vi "Process.vi"(9 "process sync":refnum<notifier>, 10 "TopLevel":refnum<class "TopLevel.lvclass">, 11 "DLP2 in":refnum<class "DLP2.lvclass">) -> ()   [LabVIEW 2022 SP3, in "DLP2.lvclass"]
doc: "Developed by Kevin Thompson\nkevin@thompsonengineering.net\n\nCopyright 2018\nThompson Engineering, LLC"
uses:
  DLP2.lvclass
  DataTypes/Read Data--cluster.ctl
  TopLevel/TopLevel.lvclass
  DataTypes/Process - AppData--cluster.ctl
  DataTypes/Settings--cluster.ctl
  DataTypes/Dependency--cluster.ctl
  Database/Database.lvclass
  DataTypes/Public Events--cluster.ctl
  Common/Controls/TD Async CmdMsg EventData--cluster.ctl
  Common/Controls/TD Sync API Event Data.ctl
  Common/Controls/APIReturnCluster--Cluster.ctl
  Common/Controls/TD Sync API Task State.ctl
  DataTypes/Images--Cluster.ctl
  <vilib>/vision/Image Controls.llb/IMAQ Image.ctl
  <vilib>/TELLC/Dynamic CVT API/TD Dynamic CVT DVR--ref.ctl
  DLP2.lvclass/DLP2.ctl
  DataTypes/PPP_Python--cluster.ctl
  TopLevel/Typedefs/PrinterHeads--Enum.ctl
  DataTypes/SeperateLayersPython--cluster.ctl
  Common/Controls/PythonVersion--Enum.ctl
  DataTypes/LoadImagesData--cluster.ctl
  Accessors/Get Settings.vi
  Accessors/Get PublicEvents.vi
  Accessors/Get Dependency.vi
  <vilib>/TELLC/SMQ/Add States to Queue using MultiLine String with vData.vi
  public/Generate Images Event.vi
  <userlib>/_OpenG.lib/file/file.llb/File Exists - Scalar__ogtk.vi
  <vilib>/vision/NI_Vision_Development_Module.lvlib
panel:
  out "Split Scale Success":bool
  out "ImageMain 3":T1(plugin-control)
  out "ImageMain 2":T1(plugin-control)
  out "DLP2ReadData":T2
  in  "Exit":bool
  # "local data monitoring"
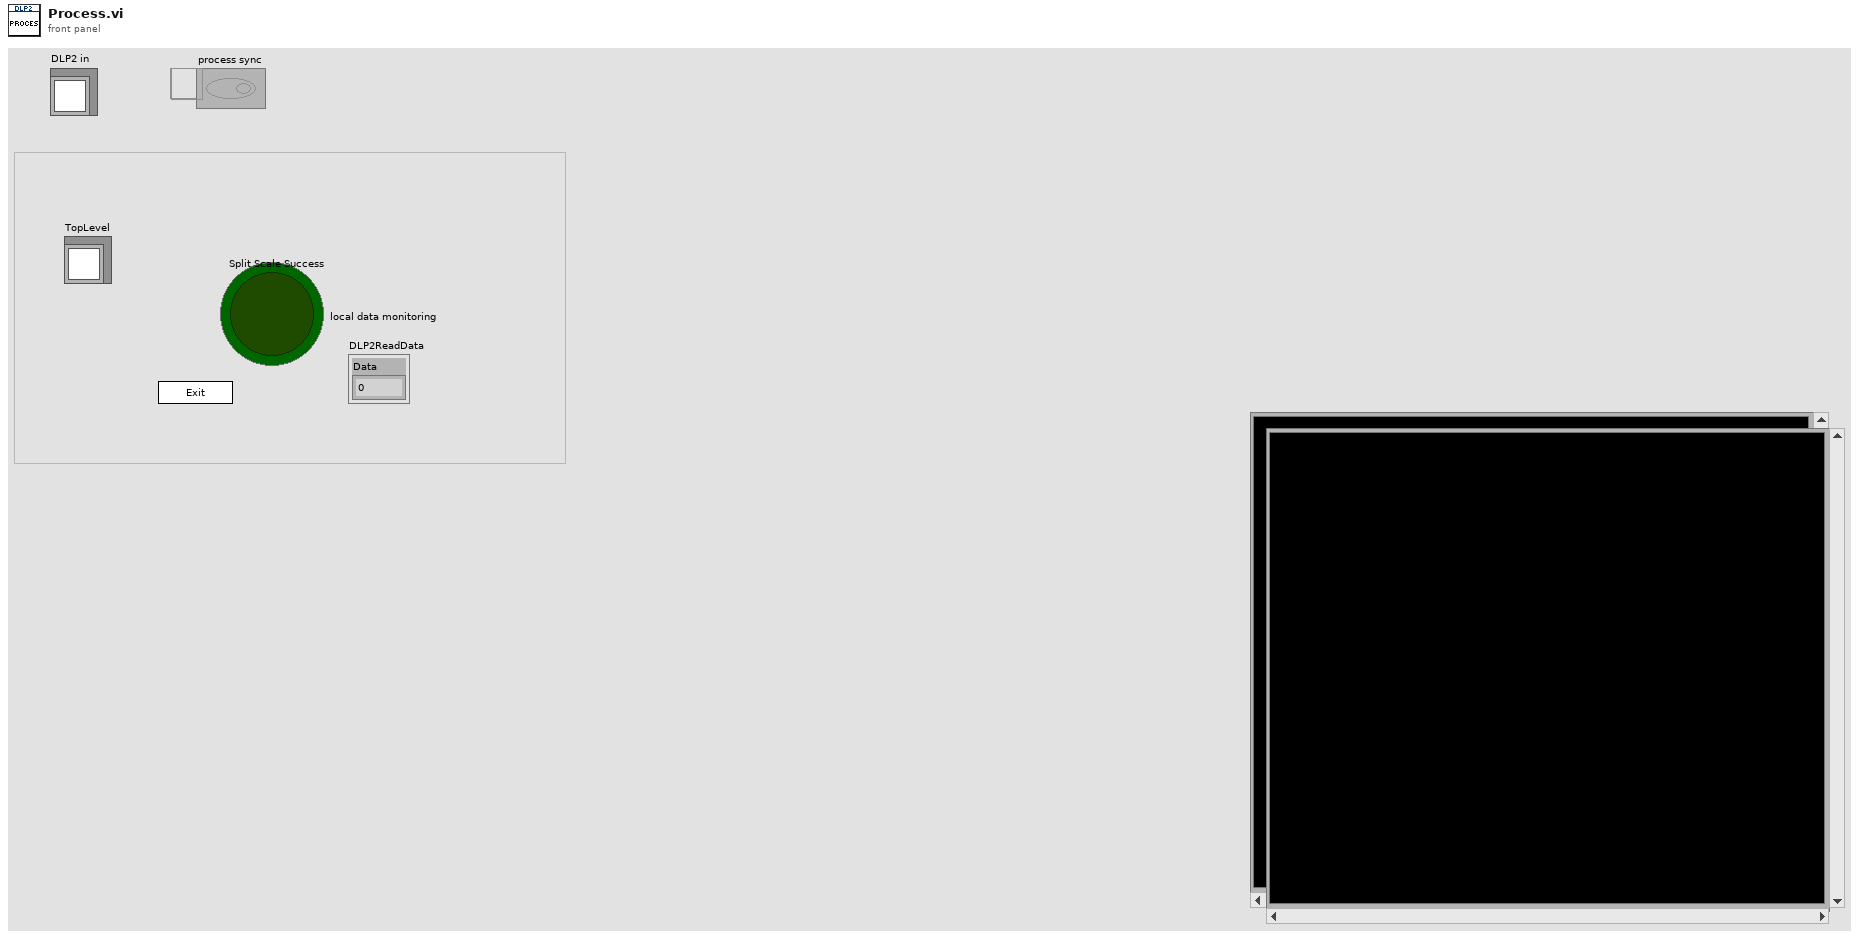
[diagram p1: front panel]
types:
  T1 = typedef "IMAQ Image.ctl" = refnum<image>
  T2 = typedef "DLP2.lvclass/Read Data--cluster.ctl" = cluster{"Data":dbl}
  T3 = typedef "DLP2.lvclass/Process - AppData--cluster.ctl" = cluster{"Core":cluster{"Current VI Reference":refnum<vi>, "Close Panel on Exit?":bool}, "SMQ":refnum<queue>, "Initialized?":bool, "Self Reference":refnum<class "DLP2.lvclass">, "Simulation?":bool, "process sync":refnum<notifier>, "vData":variant, "Settings":T4, "Dependency":T5, "Public Events":T6, "Tasks":T7[], "CuurentSyncTask":T10, "TO":i32, "Task Start ms":u32, "CurrentTaskReturnValue":variant, "DBRef":refnum<k7>, "Images":T1[], "Py session":refnum<k35>, "ConfigDict":T11}
  T4 = typedef "DLP2.lvclass/Settings--cluster.ctl" = cluster{"Simulation":bool}
  T5 = typedef "DLP2.lvclass/Dependency--cluster.ctl" = cluster{"Config":refnum<class>, "Database":refnum<class "Database.lvclass">}
  T6 = typedef "DLP2.lvclass/Public Events--cluster.ctl" = cluster{"Temp01.AsyncCmd Event":refnum<user-event>, "Temp01.AsyncMsg Event":refnum<user-event>, "stop process":refnum<user-event>, "API Incoming Event":refnum<user-event>, "API Executed Event":refnum<user-event>, "API Return Event":refnum<user-event>, "Images":refnum<user-event>}
  T7 = typedef "TD Sync API Event Data.ctl" = cluster{"Task":T8, "Command":variant, "Return Value":variant}
  T8 = typedef "APIReturnCluster--Cluster.ctl" = cluster{"Time Stamp":timestamp, "Timeout (ms)":u32, "Task State":T9, "Task Error":errorcluster, "Task ID":string, "Type":enum16{"API", "CMD"}}
  T9 = typedef "TD Sync API Task State.ctl" = enum16{"Completed", "Executing", "Errored", "Pending"}
  T10 = typedef "TD Async CmdMsg EventData--cluster.ctl" = cluster{"Time Stamp":timestamp, "CmdMsg":string, "vData":variant}
  T11 = typedef "TD Dynamic CVT DVR--ref.ctl" = refnum<data-value>
  T12 = enum32{"invalid app kind", "Development System", "Run Time System", "Student Edition", "Embedded LabVIEW", "Evaluation", "Custom"}
  T13 = enum32{"Invalid", "Standard", "Closed", "Hidden", "Minimized", "Maximized"}
  T14 = typedef "PPP_Python--cluster.ctl" = cluster{"product":string, "printer":string, "printhead":T15, "material":string, "weight":dbl, "density":dbl, "overprint":dbl, "print_wt_multiplier":dbl, "num_of_drops":i32, "gs_source":string, "gs_val_file":path, "zone_compensation":bool, "zone_comp_file":path, "bitmap":path, "save_gs_img":bool, "dithered_save_path":path, "gs_save_path":path, "rotation":bool, "driver":string, "server":string, "database":string, "user":string, "password":string}
  T15 = typedef "PrinterHeads--Enum.ctl" = enum16{"-1", "1", "2", "3", "4", "5", "6"}
  T16 = typedef "SeperateLayersPython--cluster.ctl" = cluster{"Path_to_Tiff":path, "OutputFolder":path, "DPI_x":i32, "DPI_y":i32, "Python_Version":T17}
  T17 = typedef "PythonVersion--Enum.ctl" = enum16{"3.9 64", "3.9 32", "3.12 64", "3.12 32"}
  T18 = typedef "LoadImagesData--cluster.ctl" = cluster{"Images[]":path[], "Calibration":bool, "Heads[]":u8[]}
  T19 = typedef "DLP2.lvclass/AsynCmd_Temp01--enum.ctl" = enum16{"LoadTiffImage", "SeperateLayersPython", "InvokePPP", "LoadImages"}
  T20 = enum32{"Invalid", "Standard", "Closed", "Hidden", "Minimized", "Maximized"}[]
  T21 = typedef "Image Type" = u32
  T22 = cluster{"Current VI Reference":refnum<vi>, "Close Panel on Exit?":bool}
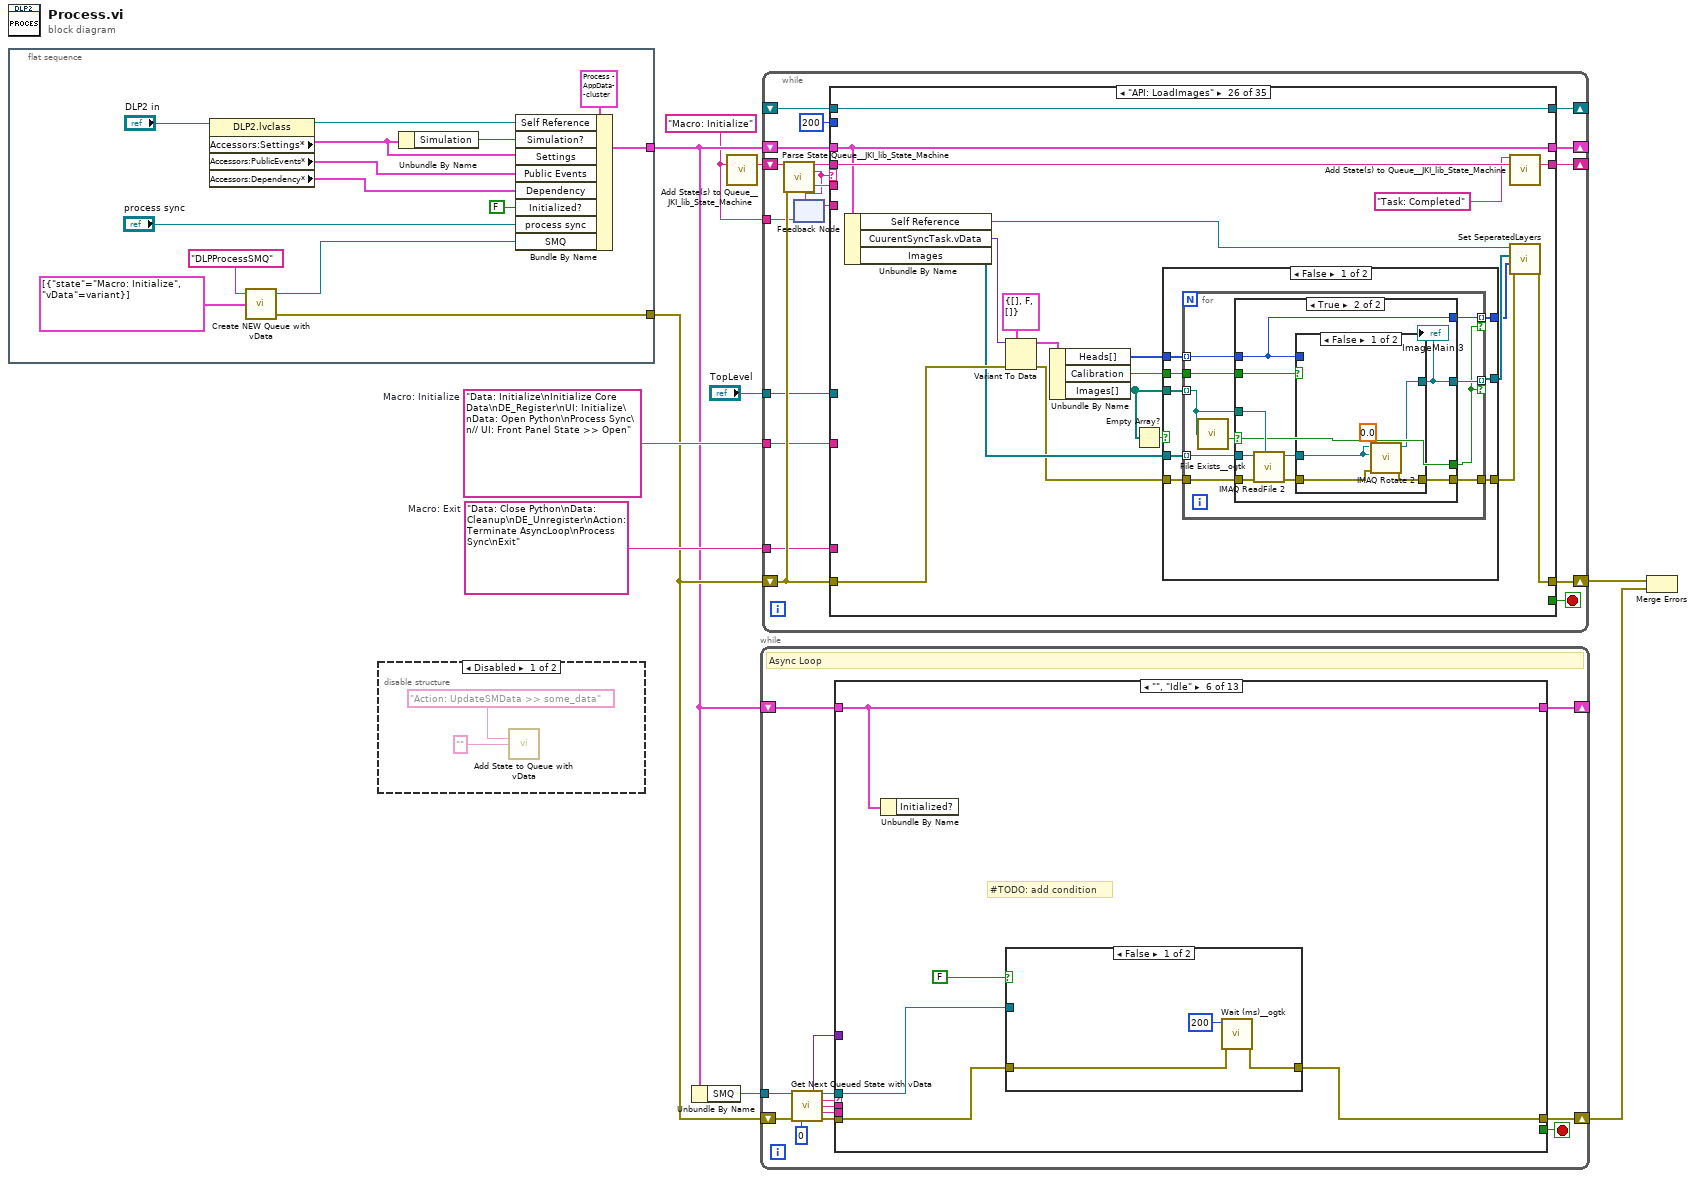
[diagram p0: block diagram]
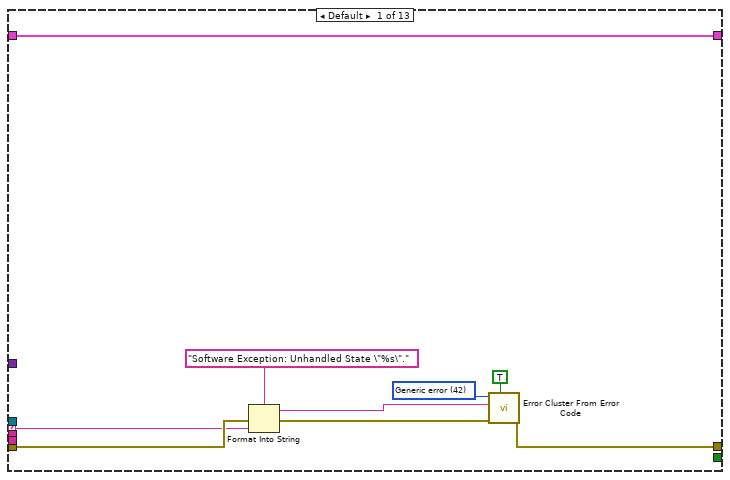
[diagram p3: hidden frame]
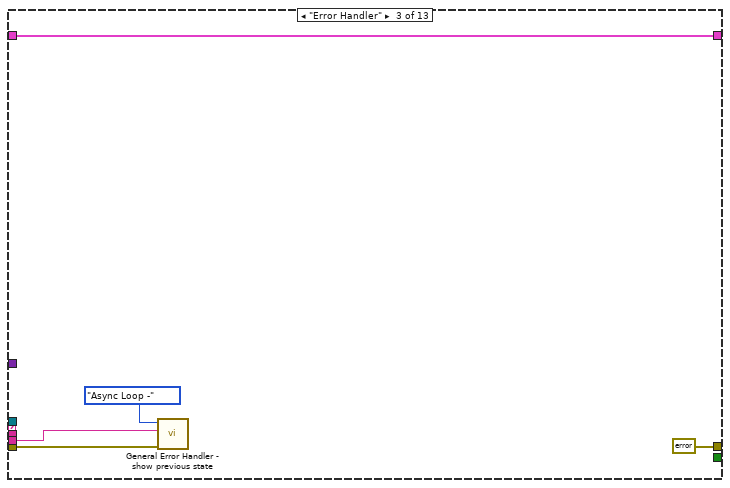
[diagram p5: hidden frame]
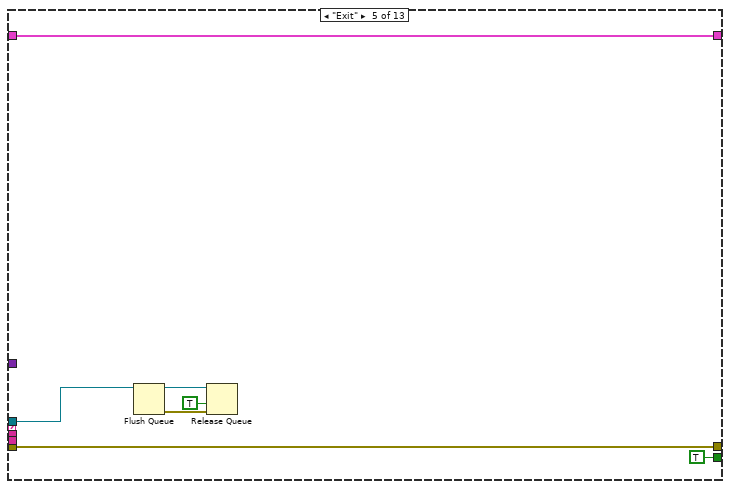
[diagram p7: hidden frame]
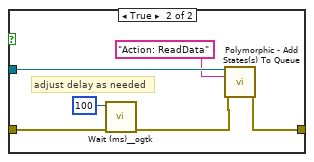
[diagram p8: hidden frame]
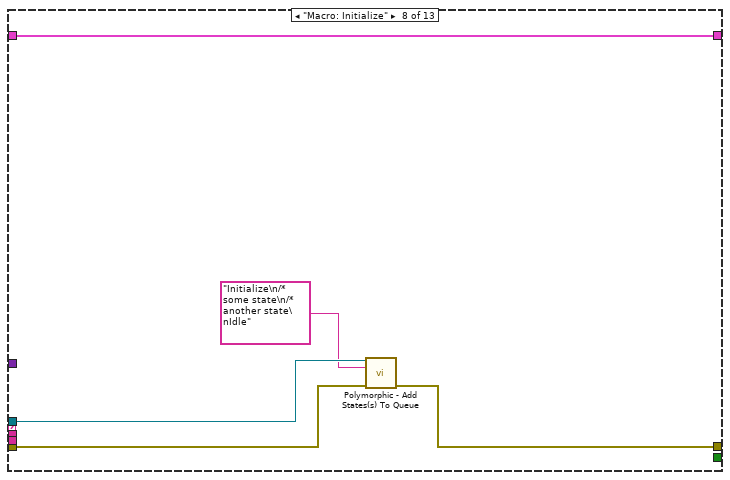
[diagram p10: hidden frame]
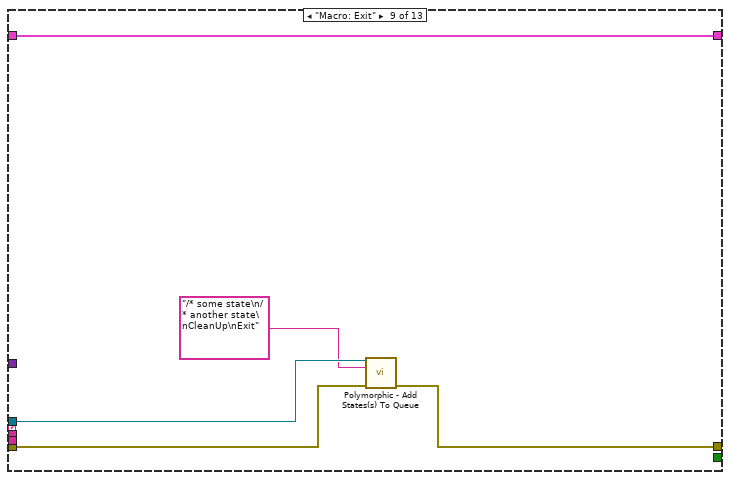
[diagram p11: hidden frame]
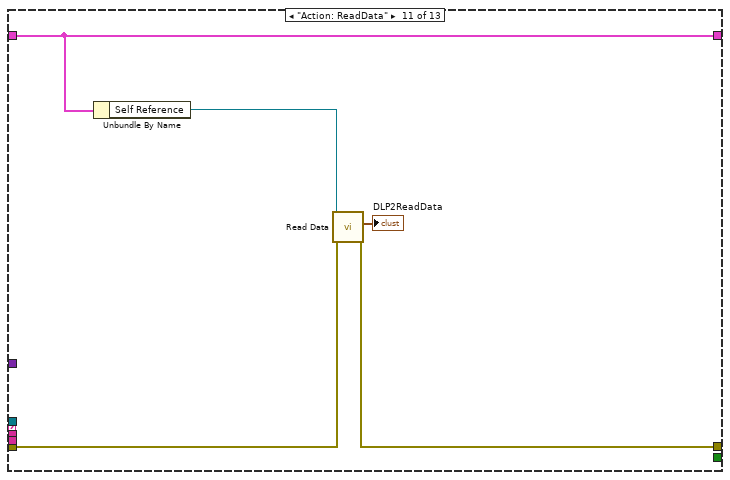
[diagram p13: hidden frame]
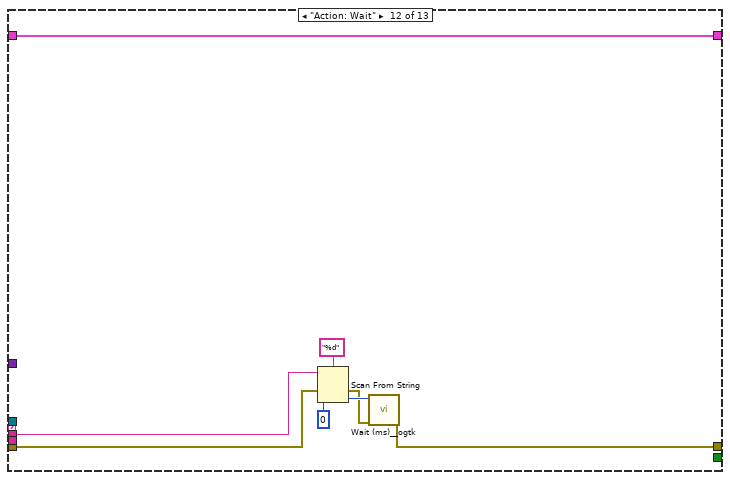
[diagram p14: hidden frame]
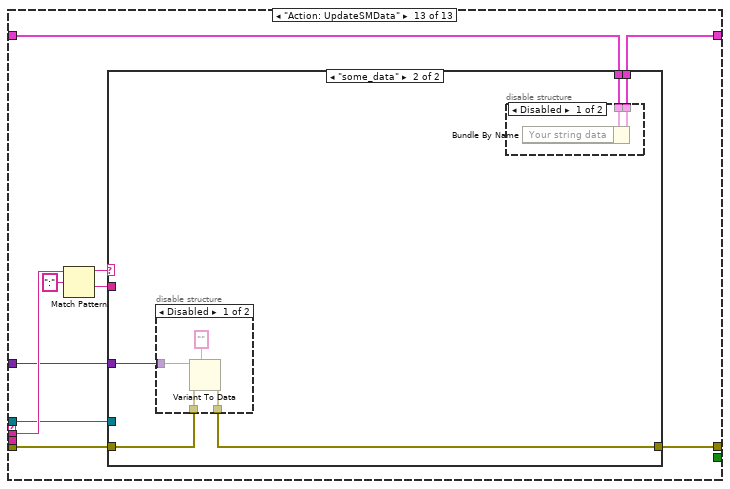
[diagram p15: hidden frame]
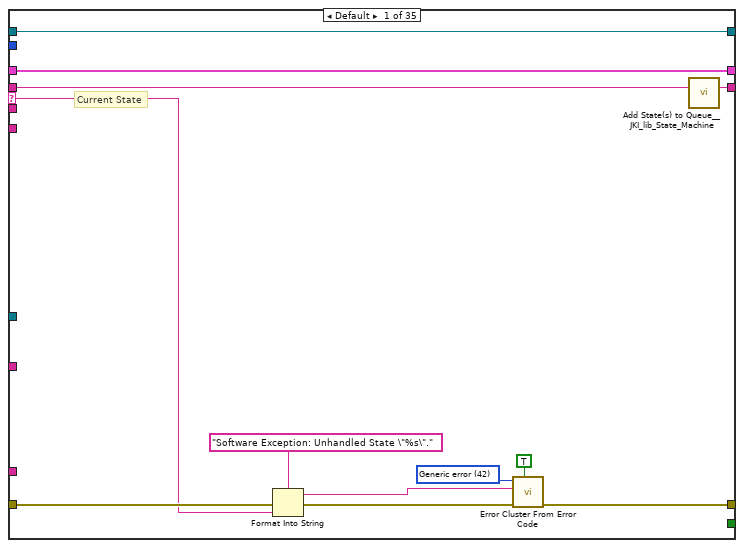
[diagram p19: hidden frame]
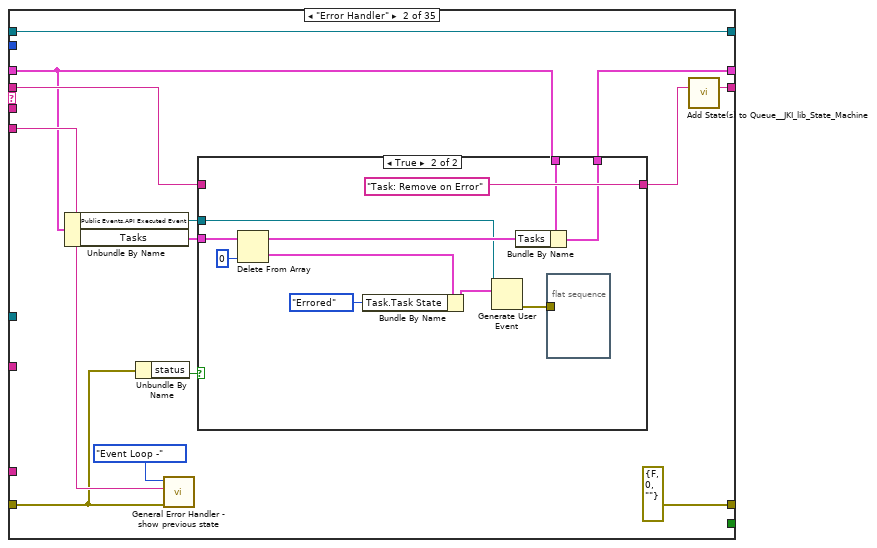
[diagram p20: hidden frame]
diagram:
  w8 = "Data: Close Python\nData: Cleanup\nDE_Unregister\nAction: Terminate AsyncLoop\nProcess Sync\nExit"  # Macro: Exit
  w9 = "Data: Initialize\nInitialize Core Data\nDE_Register\nUI: Initialize\nData: Open Python\nProcess Sync\n// UI: Front Panel State >> Open"  # Macro: Initialize
  w2 = "Macro: Initialize"
  n1 = flat-sequence {
    tunnel: [w24] -> w5
    tunnel: [w21] -> w7
    frame #0 {
      n2 = property class="DLP2.lvclass"(reference="DLP2 in") -> (reference out=w17:refnum<class "DLP2.lvclass">, "Accessors:Settings*"=w12:T4, "Accessors:PublicEvents*"=w14:T6, "Accessors:Dependency*"=w15:T5)  [unwired: 1 in, 1 out]
      n3 = call <vilib>:"Create NEW Queue with vData.vi"("Initial States"=cluster{"state":string, "vData":variant}[] [{"state"="Macro: Initialize", "vData"=variant}], "Name (SMQ)"="DLPProcessSMQ") -> ("error out"=w21:errorcluster, "queue out"=w23:refnum<queue>)  [unwired: 2 in]
      n4 = Unbundle By Name(w12) -> ("Simulation"=w13:bool)
      n5 = Bundle By Name(cluster=T3 {"Core"={"Current VI Reference"=refnum, "Close Panel on Exit?"=FALSE}, "SMQ"=refnum, "Initialized?"=FALSE, "Self Reference"=refnum, "Simulation?"=FALSE, "process sync"=refnum, "vData"=variant, "Settings"={"Simulation"=FALSE}, "Dependency"={"Config"=refnum, "Database"=refnum}, "Public Events"={"Temp01.AsyncCmd Event"=refnum, "Temp01.AsyncMsg Event"=refnum, "stop process"=refnum, "API Incoming Event"=refnum, "API Executed Event"=refnum, "API Return Event"=refnum, "Images"=refnum}, "Tasks"=[], "CuurentSyncTask"={"Time Stamp"=timestamp(0 s since 1904-01-01), "CmdMsg"="", "vData"=variant}, "TO"=0, "Task Start ms"=0, "CurrentTaskReturnValue"=variant, "DBRef"=refnum, "Images"=[], "Py session"=refnum, "ConfigDict"=refnum} ("SM2 AppData"), "Self Reference"=w17, "Simulation?"=w13, "Settings"=w12, "Public Events"=w14, "Dependency"=w15, "Initialized?"=FALSE, "process sync"="process sync", "SMQ"=w23) -> (w24:T3)
    }
  }
  n6 = disable-structure shown="Disabled" {
    frame Disabled {
      n7 = call <vilib>:"Add State to Queue with vData.vi"("state in"="Action: UpdateSMData >> some_data", "vData (\"\")"="") -> ()  [unwired: 10 in, 4 out]
    }
    frame Enabled {
    }
  }
  n8 = Unbundle By Name(w5) -> ("SMQ"=w6:refnum<queue>)
  n9 = call <vilib>:"Add State(s) to Queue__JKI_lib_State_Machine.vi"("State(s) in (\"\")"=w2) -> ("States Out"=w10:string)  [unwired: 14 in]
  n10 = while {
    shift-right: [w36] -> w3
    shift-left: w7 -> [w38]
    tunnel: w6 -> [w34]
    shift-right: [w32] -> _
    shift-left: w5 -> [w33]
    stop <- w27 stop-if-true
    # "Async Loop"
    n11 = call <vilib>:"Get Next Queued State with vData.vi"("queue in"=w34, "error in (no error)"=w38, "timeout (100)"=0) -> ("vData out"=w31:variant, "queue out"=w35:refnum<queue>, "Next State"=w39:string, "queued msg"=w29:string, "Prev State"=w28:string, "error out"=w37:errorcluster)  [unwired: 6 in, 1 out]
    n12 = case shown="\"\", \"Idle\"" w39 {
      tunnel: w35 -> [_ _ _ _ w58 w68 _ w84 w89 _ _ _ w111]
      tunnel: w29 -> [_ _ _ _ _ _ _ _ _ _ _ w100 w113]
      selector: w39 -> [w40 _ _ _ _ _ _ _ _ _ _ _ _]
      tunnel: w37 -> [w42 w50 w52 w57 w64 w66 w80 w83 w88 w92 w95 w99 w108]
      tunnel: [w41 w50 errorcluster {"status"=FALSE, "code"=0, "source"=""} ("error constant") w57 w64 w65 w80 w82 w87 w92 w94 w102 w107] -> w36
      tunnel: w33 -> [w48 w49 w55 w56 w63 w67 w79 w85 w90 w91 w97 w105 w110]
      tunnel: [w48 w49 w55 w56 w63 w67 w79 w85 w90 w91 w97 w105 w109] -> w32
      tunnel: w31 -> [_ _ _ _ _ _ _ _ _ _ _ _ w112]
      tunnel: w28 -> [_ _ w51 _ _ _ _ _ _ _ _ _ _]
      tunnel: [_ _ _ _ TRUE _ _ _ _ _ _ _ _] -> w27
      frame Default {
        w44 = 42 items=["No error", "Argument error", "Memory is full", "Out of zone", "End of file", "File already open", "Generic file I/O error", "File not found", "File permission error", "Disk is full", "Duplicate path", "Too many files open", "System feature not enabled", "Resource file not found", "Cannot add resource", "Resource not found", "Image not found", "Image memory error", "Pen does not exist", "Config type invalid", "Config token not found", "Config parse error", "Config memory error", "Bad external code format", "Bad external code offset", "External code not present", "Null window", "Destroy window error", "Null menu", "Print aborted", "Bad print record", "Print driver error", "Windows error during printing", "Memory error during printing", "Print dialog error", "Generic print error", "Invalid device refnum", "Device not found", "Device parameter error", "Device unit error", "Cannot open device", "Device call aborted", "Generic error", "Cancelled by user", "Object ID too low", "Object ID too high", "Object not in heap", "Unknown heap", "Unknown object (invalid DefProc)", "Unknown object (DefProc not in table)", "Message out of range", "Invalid (null) method", "Unknown message", "Manager call not supported", "Bad address", "Network operation in progress", "Network operation timed out", "Connection is busy", "Network attribute not supported", "Network error", "Address in use", "System out of memory", "Connection aborted", "Connection refused", "Not connected", "Already connected", "Connection closed", "Initialization error (interapplication manager)", "Bad occurrence", "Wait on unbound occurrence handler", "Occurrence queue overflow", "Datalog type conflict", "Unused", "Unrecognized type (interapplication manager)", "Memory corrupt", "Failed to make temporary DLL", "Old CIN version", "Drag socket not found", "Failed to load drop-object", "Failed to register OLE object", "Failed to release OLE object", "Format specifier type mismatch", "Unknown format specifier", "Too few format specifiers", "Too many format specifiers", "Scan failed", "Newer CIN version", "Error converting to variant", "Runtime menu error", "Password tampered", "Variant attribute not found", "Incompatible variant data type", "Event data is not available", "Event Store is not present", "Occurrence is not found", "Event Queue is not created", "Event info is not available", "Refnum passed is NULL", "Error retrieving Class GUID", "Error retrieving CoClass GUID", "Error retrieving TypeLib GUID.", "Bad built application magic bytes.", "Specific driver is different from the specific driver associated with the Logical Name.", "There is no session opened to the class driver.", "Max Error", "MAX - Error with config objects", "MAX - Error loading configuration", "MAX - Group not supported"]
        n13 = Format Into String(format string="Software Exception: Unhandled State \"%s\"." ("message"), error in=w42, w40) -> (resulting string=w45:string, error out=w46:errorcluster)  [unwired: 1 in]
        n14 = call <vilib>:"Error Cluster From Error Code.vi"("show call chain? (False)"=TRUE, "error in (no error)"=w46, "error message (\"\")"=w45, "error code (0)"=w44) -> ("error out"=w41:errorcluster)  [unwired: 5 in]
      }
      frame "Initialize" {
      }
      frame "Error Handler" {
        n15 = call "General Error Handler - show previous state.vi"("error in (no error)"=w52, "Previous State"=w51, "Loop Select"=enum16{"Event Loop -", "Async Loop -"}."Async Loop -") -> ()  [unwired: 7 in, 2 out]
      }
      frame "CleanUp" {
      }
      frame "Exit" {
        n16 = Flush Queue(queue=w58) -> (queue out=w61:refnum<queue>, error out=w60:errorcluster)  [unwired: 1 in, 1 out]
        n17 = Release Queue(queue=w61, force destroy? (F)=TRUE, error in (no error)=w60) -> ()  [unwired: 3 out]
      }
      frame "", "Idle" {
        # "#TODO: add condition"
        n18 = Unbundle By Name(w67) -> ()  [unwired: 1 out]
        n19 = case shown="False" FALSE {
          tunnel: w68 -> [_ w78]
          tunnel: w66 -> [w70 w76]
          tunnel: [w71 w73] -> w65
          frame False {
            n20 = call <userlib>:"Wait (ms)__ogtk.vi"("error in (no error)"=w70, "milliseconds to wait"=u32 200) -> ("error out"=w71:errorcluster)  [unwired: 8 in, 1 out]
          }
          frame True {
            # "adjust delay as needed"
            n21 = call <userlib>:"Wait (ms)__ogtk.vi"("error in (no error)"=w76, "milliseconds to wait"=u32 100) -> ("error out"=w75:errorcluster)  [unwired: 8 in, 1 out]
            n22 = call-poly <vilib>:"Polymorphic - Add States(s) To Queue.vi"("queue in"=w78, "state in"="Action: ReadData", "error in"=w75) -> ("error out"=w73:errorcluster)  [unwired: 9 in, 3 out]
          }
        }
      }
      frame "------ Macro ------" {
      }
      frame "Macro: Initialize" {
        n23 = call-poly <vilib>:"Polymorphic - Add States(s) To Queue.vi"("queue in"=w84, "states in"="Initialize\n/* some state\n/* another state\nIdle", "error in"=w83) -> ("error out"=w82:errorcluster)  [unwired: 10 in, 2 out]
      }
      frame "Macro: Exit" {
        n24 = call-poly <vilib>:"Polymorphic - Add States(s) To Queue.vi"("queue in"=w89, "states in"="/* some state\n/* another state\nCleanUp\nExit", "error in"=w88) -> ("error out"=w87:errorcluster)  [unwired: 10 in, 2 out]
      }
      frame "------ Action ------" {
      }
      frame "Action: ReadData" {
        n25 = Unbundle By Name(w97) -> ("Self Reference"=w96:refnum<class "DLP2.lvclass">)
        n26 = call "Read Data.vi"("error in (no error)"=w95, "DLP2 in"=w96) -> ("error out"=w94:errorcluster, "DLP2ReadData"=→"DLP2ReadData":T2)  [unwired: 7 in, 1 out]
      }
      frame "Action: Wait" {
        n27 = Scan From String(format string="%d", input string=w100, error in=w99, default 1=u32 0) -> (error out=w98:errorcluster, output 1=w104:u32)  [unwired: 1 in, 2 out]
        n28 = call <userlib>:"Wait (ms)__ogtk.vi"("error in (no error)"=w98, "milliseconds to wait"=w104) -> ("error out"=w102:errorcluster)  [unwired: 8 in, 1 out]
      }
      frame "Action: UpdateSMData" {
        n29 = Match Pattern(string=w113, regular expression=":") -> (before substring=w115:string, after substring=w106:string)  [unwired: 1 in, 2 out]
        n30 = case shown="\"some_data\"" w115 {
          tunnel: w112 -> [_ w122]
          tunnel: w111 -> [_ _]
          tunnel: w110 -> [w116 w121]
          tunnel: [w116 w120] -> w109
          tunnel: w108 -> [w117 w119]
          tunnel: [w117 w118] -> w107
          tunnel: w106 -> [_ _]
          frame Default {
            # "#NOTE:\noptionally add error here."
          }
          frame "some_data" {
            n31 = disable-structure shown="Disabled" {
              disable-tunnel: w122 -> [w129 _]
              disable-tunnel: w119 -> [w127 w130]
              disable-tunnel: [w126 w130] -> w118
              frame Disabled {
                n32 = Variant To Data(error in=w127, type="", Variant=w129) -> (error out=w126:errorcluster)  [unwired: 1 out]
              }
              frame Enabled {
              }
            }
            n33 = disable-structure shown="Disabled" {
              disable-tunnel: w121 -> [w124 w125]
              disable-tunnel: [w123 w125] -> w120
              frame Disabled {
                n34 = Bundle By Name(cluster=w124) -> (w123:T3)  [unwired: 1 in]
              }
              frame Enabled {
              }
            }
          }
        }
      }
    }
  }
  n35 = while {
    shift-right: [w142] -> _
    shift-left: w5 -> [w141]
    shift-right: [w145] -> w4
    shift-left: w7 -> [w140]
    shift-right: [w144] -> _
    shift-left: w10 -> [w146]
    shift-right: [w139] -> _
    shift-left: _ -> [w138]
    tunnel: w9 -> [w136]
    tunnel: w8 -> [w135]
    tunnel: w2 -> [w134]
    tunnel: "TopLevel" -> [w131]
    stop <- w143 stop-if-true
    n36 = call <vilib>:"Parse State Queue__JKI_lib_State_Machine.vi"("State Queue"=w146, "Error In (no error)"=w140) -> ("Remaining States"=w148:string, "Current State"=w133:string, "Arguments"=w147:string)  [unwired: 11 in]
    n37 = feedback #1(w134) -> (w132:string)
    n38 = feedback-in #1(w133) -> ()
    n39 = case shown="\"API: LoadImages\"" w133 {
      selector: w133 -> [w150 _ _ _ _ _ _ _ _ _ _ _ _ _ _ _ _ _ _ _ _ _ _ _ _ _ _ _ _ _ _ _ _ _ _]
      tunnel: w148 -> [w154 w164 w192 w200 w347 w362 w370 w375 w379 w384 w391 w403 w418 w425 w430 w438 w447 w459 w486 w492 w503 w508 w513 w529 w558 w608 w667 w672 w683 w692 w697 w708 w727 w755 w782]
      tunnel: w147 -> [_ _ _ _ _ _ _ _ _ _ _ _ _ _ _ _ w442 w453 _ _ _ _ _ _ _ _ _ _ w673 _ _ _ _ _ _]
      tunnel: w141 -> [w152 w162 w190 w198 w344 w355 w367 w372 w378 w381 w388 w401 w413 w420 w427 w433 w445 w455 w483 w489 w500 w505 w510 w518 w550 w603 w663 w669 w681 w689 w694 w699 w717 w747 w775]
      tunnel: [w156 errorcluster {"status"=FALSE, "code"=0, "source"=""} ("error out") w189 w197 w345 w359 w363 w373 w376 w382 w386 w397 w407 w421 w428 w434 w443 w456 w484 w490 w501 w506 w511 w521 w538 w595 w658 w670 w674 w684 w695 w703 w720 w746 w774] -> w145
      tunnel: w140 -> [w155 w161 w189 w196 w345 w359 w364 _ w376 w382 w385 w393 w406 w422 w428 w435 w444 w457 w484 w490 w501 w506 w511 w524 w552 w604 w661 w670 w675 w685 w695 w702 w719 w745 w773]
      tunnel: [w153 w173 w191 w199 w346 w361 w369 w375 w379 w383 w390 w402 w417 w424 w429 w437 w446 w458 w485 w491 w502 w507 w512 w528 w557 w607 w666 w671 w682 w691 w696 w707 w726 w754 w781] -> w144
      tunnel: [_ _ TRUE _ _ _ _ _ _ _ _ _ _ _ _ _ _ _ _ _ _ _ _ _ _ _ _ _ _ _ _ _ _ _ _] -> w143
      tunnel: [w152 w163 w190 w195 w344 w360 w367 w372 w378 w381 w388 w399 w415 w420 w427 w433 w445 w455 w483 w489 w500 w505 w510 w519 w551 w603 w660 w669 w681 w689 w694 w700 w718 w747 w775] -> w142
      tunnel: [w149 w171 w187 w193 w343 w352 w368 w374 w377 w380 w389 w400 w414 w419 w426 w436 w441 w452 w482 w488 w494 w504 w509 w527 w556 w606 w665 w668 w680 w690 w693 w706 w725 w753 w780] -> w139
      tunnel: w138 -> [w149 w171 w187 w193 w343 w352 w368 _ w377 w380 w389 w400 w414 w419 w426 w436 w441 w452 w482 w488 w494 w504 w509 w527 w556 w606 w665 w668 w680 w690 w693 w706 w725 w753 w780]
      tunnel: 200 ("Timeout") -> [_ _ _ w194 _ _ _ _ _ _ _ _ _ _ _ _ _ _ _ _ _ _ _ _ _ _ _ _ _ _ _ _ _ _ _]
      tunnel: w136 -> [_ _ _ _ _ _ _ _ _ _ _ _ _ _ _ _ _ _ _ w487 _ _ _ _ _ _ _ _ _ _ _ _ _ _ _]
      tunnel: w135 -> [_ _ _ _ _ _ _ _ _ _ _ _ _ _ _ _ _ _ _ _ w493 _ _ _ _ _ _ _ _ _ _ _ _ _ _]
      tunnel: w132 -> [_ w169 _ _ _ _ _ _ _ _ _ _ _ _ _ _ _ _ _ _ _ _ _ _ _ _ _ _ _ _ _ _ _ _ _]
      tunnel: w131 -> [_ _ _ _ _ _ _ _ _ _ _ _ w405 _ _ _ _ _ _ _ _ _ _ _ _ _ _ _ _ _ _ _ _ _ _]
      frame Default {
        w159 = 42 items=["No error", "Argument error", "Memory is full", "Out of zone", "End of file", "File already open", "Generic file I/O error", "File not found", "File permission error", "Disk is full", "Duplicate path", "Too many files open", "System feature not enabled", "Resource file not found", "Cannot add resource", "Resource not found", "Image not found", "Image memory error", "Pen does not exist", "Config type invalid", "Config token not found", "Config parse error", "Config memory error", "Bad external code format", "Bad external code offset", "External code not present", "Null window", "Destroy window error", "Null menu", "Print aborted", "Bad print record", "Print driver error", "Windows error during printing", "Memory error during printing", "Print dialog error", "Generic print error", "Invalid device refnum", "Device not found", "Device parameter error", "Device unit error", "Cannot open device", "Device call aborted", "Generic error", "Cancelled by user", "Object ID too low", "Object ID too high", "Object not in heap", "Unknown heap", "Unknown object (invalid DefProc)", "Unknown object (DefProc not in table)", "Message out of range", "Invalid (null) method", "Unknown message", "Manager call not supported", "Bad address", "Network operation in progress", "Network operation timed out", "Connection is busy", "Network attribute not supported", "Network error", "Address in use", "System out of memory", "Connection aborted", "Connection refused", "Not connected", "Already connected", "Connection closed", "Initialization error (interapplication manager)", "Bad occurrence", "Wait on unbound occurrence handler", "Occurrence queue overflow", "Datalog type conflict", "Unused", "Unrecognized type (interapplication manager)", "Memory corrupt", "Failed to make temporary DLL", "Old CIN version", "Drag socket not found", "Failed to load drop-object", "Failed to register OLE object", "Failed to release OLE object", "Format specifier type mismatch", "Unknown format specifier", "Too few format specifiers", "Too many format specifiers", "Scan failed", "Newer CIN version", "Error converting to variant", "Runtime menu error", "Password tampered", "Variant attribute not found", "Incompatible variant data type", "Event data is not available", "Event Store is not present", "Occurrence is not found", "Event Queue is not created", "Event info is not available", "Refnum passed is NULL", "Error retrieving Class GUID", "Error retrieving CoClass GUID", "Error retrieving TypeLib GUID.", "Bad built application magic bytes.", "Specific driver is different from the specific driver associated with the Logical Name.", "There is no session opened to the class driver.", "Max Error", "MAX - Error with config objects", "MAX - Error loading configuration", "MAX - Group not supported"]
        # "Current State"
        n40 = Format Into String(format string="Software Exception: Unhandled State \"%s\"." ("message"), error in=w155, w150) -> (resulting string=w158:string, error out=w157:errorcluster)  [unwired: 1 in]
        n41 = call <vilib>:"Error Cluster From Error Code.vi"("show call chain? (False)"=TRUE, "error in (no error)"=w157, "error message (\"\")"=w158, "error code (0)"=w159) -> ("error out"=w156:errorcluster)  [unwired: 5 in]
        n42 = call <vilib>:"Add State(s) to Queue__JKI_lib_State_Machine.vi"("State(s) in (\"\")"=w154) -> ("States Out"=w153:string)  [unwired: 14 in]
      }
      frame "Error Handler" {
        n43 = Unbundle By Name(w162) -> ("Public Events.API Executed Event"=w168:refnum<user-event>, "Tasks"=w167:T7[])
        n44 = Unbundle By Name(w161) -> ("status"=w166:bool)
        n45 = call "General Error Handler - show previous state.vi"("error in (no error)"=w161, "Previous State"=w169, "Loop Select"=enum16{"Event Loop -", "Async Loop -"}."Event Loop -") -> ()  [unwired: 7 in, 2 out]
        n46 = case shown="True" w166 {
          tunnel: w164 -> [w175 _]
          tunnel: [w175 "Task: Remove on Error"] -> w165
          tunnel: w167 -> [_ w186]
          tunnel: w162 -> [w174 w183]
          tunnel: [w174 w182] -> w163
          tunnel: w168 -> [_ w179]
          frame False {
          }
          frame True {
            n47 = Delete From Array(array=w186, index=0) -> (deleted portion=w178:T7, array with subset deleted=w181:T7[])  [unwired: 1 in]
            n48 = Bundle By Name(cluster=w178, "Task.Task State"=TD_Sync_API_Task_State."Errored") -> (w180:T7)
            n49 = Generate User Event(user event=w179, event data cluster=w180) -> (error out=w176:errorcluster)  [unwired: 2 in, 1 out]
            n50 = Bundle By Name(cluster=w183, "Tasks"=w181) -> (w182:T3)
            n51 = flat-sequence {
              tunnel: w176 -> [_]
              frame #0 {
              }
            }
          }
        }
        n52 = call <vilib>:"Add State(s) to Queue__JKI_lib_State_Machine.vi"("State(s) in (\"\")"=w165) -> ("States Out"=w173:string)  [unwired: 14 in]
      }
      frame "Exit" {
        n53 = call <vilib>:"Add State(s) to Queue__JKI_lib_State_Machine.vi"("State(s) in (\"\")"=w192) -> ("States Out"=w191:string)  [unwired: 14 in]
      }
      frame "", "Event Structure", "Idle" {
        n54 = event shown="[2] <Public Events.API Executed Event>: User Event" {
          selector: w193 -> [_ _ _ _ _ _ _ _]
          dyn-events: _ -> [_ _ _ _ _ _ _ _]
          timeout: w194 -> [_ _ _ _ _ _ _ _]
          tunnel: w200 -> [w204 w221 w277 w297 w303 w306 w313 w329]
          tunnel: [w203 w220 w276 w296 w302 w305 w312 w328] -> w199
          tunnel: w198 -> [w201 w207 w266 w294 w300 w308 w316 w318]
          tunnel: [w202 w205 w252 w295 w301 w309 w317 w326] -> w197
          tunnel: w196 -> [w202 w205 w251 w295 w301 w309 w317 w325]
          tunnel: [w201 w208 w267 w294 w300 w308 w315 w320] -> w195
          event Timeout {
            n55 = event-data() -> ()  [unwired: 1 in, 1 out]
            n56 = call <vilib>:"Add State(s) to Queue__JKI_lib_State_Machine.vi"("State(s) in (\"\")"=w204) -> ("States Out"=w203:string)  [unwired: 14 in]
          }
          event User Event {
            n57 = event-data() -> ("Task"=w215:T8, "Command"=w214:variant)  [unwired: 1 in, 5 out]
            n58 = Unbundle By Name(w207) -> ("Tasks"=w210:T7[])
            n59 = Bundle By Name(cluster=T7 {"Task"={"Time Stamp"=timestamp(0 s since 1904-01-01), "Timeout (ms)"=0, "Task State"=enum."Completed", "Task Error"={"status"=FALSE, "code"=0, "source"=""}, "Task ID"="", "Type"=enum."API"}, "Command"=variant, "Return Value"=variant} ("API Event Data"), "Task"=w215, "Command"=w214) -> (w209:T7)
            n60 = Unbundle By Name(w209) -> ("Task.Task ID"=w219:string)
            n61 = String Subset(string=w219, length (rest)=4 ("length (rest)")) -> (substring=w217:string)  [unwired: 1 in]
            n62 = Empty Array?(array=w210) -> (empty?=w211:bool)
            n63 = Equal?(x=w217, y="DLP2") -> (x = y?=w212:bool)
            n64 = case shown="True" w212 {
              tunnel: w211 -> [_ w227]
              tunnel: w210 -> [_ w229]
              tunnel: w209 -> [_ w228]
              tunnel: w207 -> [w222 w226]
              tunnel: [w222 w225] -> w208
              tunnel: [_ w224] -> w206
              tunnel: w205 -> [_ w223]
              frame False {
              }
              frame True {
                n65 = case shown="False" w227 {
                  tunnel: w229 -> [w233 w246]
                  tunnel: w228 -> [w232 w244]
                  tunnel: w226 -> [w231 w242]
                  tunnel: [w230 w241] -> w225
                  tunnel: [_ w237] -> w224
                  tunnel: w223 -> [_ w235]
                  frame False {
                    n66 = Build Array (concatenate)(w233, w232) -> (w234:T7[])
                    n67 = Bundle By Name(cluster=w231, "Tasks"=w234) -> (w230:T3)
                  }
                  frame True {
                    n68 = Unbundle By Name(w244) -> ("Command"=w245:variant)
                    n69 = Build Array (concatenate)(w246, w244) -> (w247:T7[])
                    n70 = Tick Count (ms)() -> (millisecond timer value=w248:u32)
                    n71 = Variant To Data(error in=w235, type=T10 {"Time Stamp"=timestamp(0 s since 1904-01-01), "CmdMsg"="", "vData"=variant} ("Async EvData"), Variant=w245) -> (data=w240:T10, error out=w236:errorcluster)
                    n72 = Unbundle By Name(w240) -> ("CmdMsg"=w238:string)
                    n73 = Bundle By Name(cluster=w242, "TO"=100, "Tasks"=w247, "Task Start ms"=w248, "CuurentSyncTask"=w240) -> (w241:T3)
                    n74 = Format Into String(format string="API: %s", error in=w236, w238) -> (resulting string=w237:string)  [unwired: 1 in, 1 out]
                  }
                }
              }
            }
            n75 = call <vilib>:"Add State(s) to Queue__JKI_lib_State_Machine.vi"("State(s) in Front (\"\")"=w206, "State(s) in (\"\")"=w221) -> ("States Out"=w220:string)  [unwired: 13 in]
          }
          event User Event {
            n76 = event-data() -> ("Task"=w257:T8, "Command"=w271:variant, "Return Value"=w253:variant)  [unwired: 1 in, 4 out]
            n77 = Unbundle By Name(w266) -> ("Public Events.API Return Event"=w254:refnum<user-event>, "Tasks"=w258:T7[])
            n78 = Bundle By Name(cluster=T7 {"Task"={"Time Stamp"=timestamp(0 s since 1904-01-01), "Timeout (ms)"=0, "Task State"=enum."Completed", "Task Error"={"status"=FALSE, "code"=0, "source"=""}, "Task ID"="", "Type"=enum."API"}, "Command"=variant, "Return Value"=variant} ("API Event Data"), "Task"=w257, "Command"=w271, "Return Value"=w253) -> (w268:T7)
            n79 = Delete From Array(array=w258, index=0) -> (deleted portion=w262:T7, array with subset deleted=w256:T7[])  [unwired: 1 in]
            n80 = Unbundle By Name(w268) -> ("Task.Task ID"=w275:string)
            n81 = Unbundle By Name(w262) -> ("Task.Task ID"=w263:string)
            n82 = Unbundle By Name(w257) -> ("Task ID"=w264:string, "Task State"=w255:T9)
            n83 = Empty Array?(array=w258) -> (empty?=w269:bool)
            n84 = String Subset(string=w275, length (rest)=4 ("length (rest)")) -> (substring=w273:string)  [unwired: 1 in]
            n85 = Equal?(x=w263, y=w264) -> (x = y?=w265:bool)
            n86 = Equal?(x=w273, y="DLP2") -> (x = y?=w260:bool)
            n87 = And(x=w265, y=w260) -> (x .and. y?=w259:bool)
            n88 = case shown="True" w259 {
              tunnel: w269 -> [_ _]
              tunnel: w268 -> [_ w280]
              tunnel: w266 -> [w279 w284]
              tunnel: [w279 w283] -> w267
              tunnel: w256 -> [_ w282]
              tunnel: w255 -> [_ w289]
              tunnel: w254 -> [_ w287]
              tunnel: w251 -> [w278 w286]
              tunnel: [w278 w285] -> w252
              tunnel: [_ w281] -> w250
              frame False {
              }
              frame True {
                n89 = Equal?(x=w289, y=TD_Sync_API_Task_State."Errored") -> (x = y?=w292:bool)
                n90 = Select(t="Task: Remove on Error", s=w292, f="Task: Check Pending") -> (s? t:f=w281:string)
                n91 = Bundle By Name(cluster=w284, "Tasks"=w282) -> (w283:T3)
                n92 = Generate User Event(user event=w287, event data cluster=w280, error in=w286) -> (error out=w285:errorcluster)  [unwired: 1 in, 1 out]
              }
            }
            n93 = call <vilib>:"Add State(s) to Queue__JKI_lib_State_Machine.vi"("State(s) in Front (\"\")"=w250, "State(s) in (\"\")"=w277) -> ("States Out"=w276:string)  [unwired: 13 in]
          }
          event "Exit": Value Change {
            n94 = event-data() -> ()  [unwired: 1 in, 1 out]
            n95 = call <vilib>:"Add State(s) to Queue__JKI_lib_State_Machine.vi"("State(s) in Front (\"\")"="Macro: Exit", "State(s) in (\"\")"=w297) -> ("States Out"=w296:string)  [unwired: 13 in]
          }
          event Panel Close? {
            n96 = event-data() -> ()  [unwired: 1 in, 1 out]
            n97 = event-data("Discard?"=TRUE) -> ()  [unwired: 1 in, 1 out]
            n98 = call <vilib>:"Add State(s) to Queue__JKI_lib_State_Machine.vi"("State(s) in Front (\"\")"="Macro: Exit", "State(s) in (\"\")"=w303) -> ("States Out"=w302:string)  [unwired: 13 in]
          }
          event Menu Selection (User) {
            n99 = event-data() -> ("ItemTag"=w307:string)  [unwired: 1 in, 2 out]
            n100 = case shown="\"False\", Default" w307 {
              tunnel: [""] -> w304
              frame "False", Default {
              }
            }
            n101 = call <vilib>:"Add State(s) to Queue__JKI_lib_State_Machine.vi"("State(s) in Front (\"\")"=w304, "State(s) in (\"\")"=w306) -> ("States Out"=w305:string)  [unwired: 13 in]
          }
          event User Event {
            n102 = event-data() -> ("notifier out"=w314:refnum<notifier>)  [unwired: 1 in]
            n103 = Bundle By Name(cluster=w316, "process sync"=w314) -> (w315:T3)
            n104 = call <vilib>:"Add State(s) to Queue__JKI_lib_State_Machine.vi"("State(s) in Front (\"\")"="Macro: Exit", "State(s) in (\"\")"=w313) -> ("States Out"=w312:string)  [unwired: 13 in]
          }
          event User Event {
            n105 = event-data() -> ("CmdMsg"=w323:string, "vData"=w327:variant)  [unwired: 1 in, 1 out]
            n106 = Unbundle By Name(w318) -> ("Self Reference"=w319:refnum<class "DLP2.lvclass">)
            n107 = call "get async cmd.vi"("error in (no error)"=w325, "Cmd String in"=w323) -> ("error out"=w324:errorcluster, "AsyncCmd"=w322:T19)  [unwired: 8 in]
            n108 = case shown="Default" w322 {
              tunnel: w327 -> [_ w338]
              tunnel: w324 -> [w330 w337]
              tunnel: [w330 w336] -> w326
              tunnel: [_ ""] -> w321
              tunnel: w318 -> [w331 w334]
              tunnel: [w331 w333] -> w320
              tunnel: w319 -> [_ _]
              tunnel: w318 -> [_ _]
              frame Default {
              }
              frame "LoadTiffImage" {
                n109 = disable-structure shown="Disabled" {
                  disable-tunnel: w338 -> [w341 _]
                  disable-tunnel: w337 -> [w340 w342]
                  disable-tunnel: [w339 w342] -> w336
                  frame Disabled {
                    n110 = Variant To Data(error in=w340, Variant=w341) -> (error out=w339:errorcluster)  [unwired: 1 in, 1 out]
                  }
                  frame Enabled {
                  }
                }
                n111 = Bundle By Name(cluster=w334, "vData"=variant) -> (w333:T3)
              }
            }
            n112 = call <vilib>:"Add State(s) to Queue__JKI_lib_State_Machine.vi"("State(s) in Front (\"\")"=w321, "State(s) in (\"\")"=w329) -> ("States Out"=w328:string)  [unwired: 13 in]
          }
        }
      }
      frame "---------- Core ----------" {
        n113 = call <vilib>:"Add State(s) to Queue__JKI_lib_State_Machine.vi"("State(s) in (\"\")"=w347) -> ("States Out"=w346:string)  [unwired: 14 in]
      }
      frame "Initialize Core Data" {
        w350 = T20 [enum."Closed", enum."Hidden", enum."Invalid"] items=["Invalid", "Standard", "Closed", "Hidden", "Minimized", "Maximized"]
        # "originally closed?"
        # "exe?"
        n114 = property class="App"() -> ("App.Kind"=w358:T12)  [unwired: 2 in, 2 out]
        n115 = control-ref of="Current VI Reference"() -> (w353:refnum<vi>)
        n116 = property class="VI"() -> ("FP.State"=w351:T13)  [unwired: 2 in, 2 out]
        n117 = Search 1D Array(1D array=w350, element=w351) -> (index of element=w349:i32)  [unwired: 1 in]
        n118 = Equal?(x=w358, y=T12."Run Time System" ("Application:Kind")) -> (x = y?=w356:bool)
        n119 = Greater Than 0?(x=w349) -> (x > 0?=w348:bool)
        n120 = Or(x=w348, y=w356) -> (x .or. y?=w354:bool)
        n121 = Bundle By Name(cluster=w355, "Core.Current VI Reference"=w353, "Core.Close Panel on Exit?"=w354) -> (w360:T3)
        n122 = call <vilib>:"Add State(s) to Queue__JKI_lib_State_Machine.vi"("State(s) in (\"\")"=w362) -> ("States Out"=w361:string)  [unwired: 14 in]
      }
      frame "Process Sync" {
        n123 = Unbundle By Name(w367) -> ("process sync"=w366:refnum<notifier>)
        n124 = Send Notification(notification=TRUE, notifier=w366, error in (no error)=w364) -> (error out=w363:errorcluster)  [unwired: 1 out]
        n125 = call <vilib>:"Add State(s) to Queue__JKI_lib_State_Machine.vi"("State(s) in (\"\")"=w370) -> ("States Out"=w369:string)  [unwired: 14 in]
      }
      frame "DE_Register" {
        n126 = Unbundle By Name(w372) -> ("Public Events"=w371:T6)
        n127 = register-events(w371) -> (reference out=w374:refnum<event-registration>, error out=w373:errorcluster)  [unwired: 2 in]
      }
      frame "DE_Unregister" {
        n128 = Unregister For Events(event registration refnum=w377, error in=w376) -> ()  [unwired: 1 out]
      }
      frame "---------- Data ----------" {
        n129 = call <vilib>:"Add State(s) to Queue__JKI_lib_State_Machine.vi"("State(s) in (\"\")"=w384) -> ("States Out"=w383:string)  [unwired: 14 in]
      }
      frame "Data: Close Python" {
        n130 = Unbundle By Name(w388) -> ("Py session"=w387:refnum<k35>)
        n131 = Close Python Session(session in=w387, error in=w385) -> (11:w386:errorcluster)
        n132 = call <vilib>:"Add State(s) to Queue__JKI_lib_State_Machine.vi"("State(s) in (\"\")"=w391) -> ("States Out"=w390:string)  [unwired: 14 in]
      }
      frame "Data: Open Python" {
        w392 = "3.12" ("Python Rev Key")
        n133 = call "Get Python Path.vi"("error in (no error)"=w393, "Python Rev Key"=w392) -> ("error out"=w394:errorcluster, "Python.exe path"=w396:string)  [unwired: 8 in]
        n134 = String To Path(string=w396) -> (path=w395:path)
        n135 = Open Python Session(python version=w392, python path=w395, 3:w394) -> (session out=w398:refnum<k35>, error out=w397:errorcluster)
        n136 = Bundle By Name(cluster=w401, "Py session"=w398) -> (w399:T3)
        n137 = call <vilib>:"Add State(s) to Queue__JKI_lib_State_Machine.vi"("State(s) in (\"\")"=w403) -> ("States Out"=w402:string)  [unwired: 14 in]
      }
      frame "Data: Initialize" {
        w410 = T21[] [0, 0, 0, 0, 0, 0] items=["Grayscale (U8)", "Grayscale (I16)", "Grayscale (SGL)", "Complex (CSG)", "RGB (U32)", "HSL (U32)", "RGB (U64)", "Grayscale (U16)"]
        w411 = refnum<k7> refnum  # DBRef
        w412 = T7[] []  # Tasks
        w416 = T22 {"Current VI Reference"=refnum, "Close Panel on Exit?"=FALSE}  # Core
        n138 = property class="TopLevel.lvclass"(reference=w405) -> ("Methods:Accessors:ConfigDict"=w404:T11)  [unwired: 1 in, 2 out]
        n139 = Unbundle By Name(w413) -> ()  [unwired: 1 out]
        n140 = call "CreateImages.vi"("error in (no error)"=w406, "Array 3"=w410, "Array in"=string[] ["Image1", "Image2", "Image3", "Image4", "Image5", "Image6"]) -> ("error in (no error) 2"=w407:errorcluster, "Array out"=w408:T1[])  [unwired: 7 in]
        n141 = Bundle By Name(cluster=w413, "Core"=w416, "Tasks"=w412, "DBRef"=w411, "Images"=w408, "ConfigDict"=w404) -> (w415:T3)
        n142 = call <vilib>:"Add State(s) to Queue__JKI_lib_State_Machine.vi"("State(s) in (\"\")"=w418) -> ("States Out"=w417:string)  [unwired: 14 in]
      }
      frame "Data: Cleanup" {
        n143 = Unbundle By Name(w420) -> ("Core.Current VI Reference"=w423:refnum<vi>)
        n144 = Close Reference(reference=w423, error in (no error)=w422) -> (error out=w421:errorcluster)
        n145 = call <vilib>:"Add State(s) to Queue__JKI_lib_State_Machine.vi"("State(s) in (\"\")"=w425) -> ("States Out"=w424:string)  [unwired: 14 in]
      }
      frame "---------- UI ----------" {
        n146 = call <vilib>:"Add State(s) to Queue__JKI_lib_State_Machine.vi"("State(s) in (\"\")"=w430) -> ("States Out"=w429:string)  [unwired: 14 in]
      }
      frame "UI: Initialize" {
        n147 = Unbundle By Name(w433) -> ("Core.Current VI Reference"=w432:refnum<vi>)
        n148 = call <userlib>:"Fit VI window to Largest Dec__ogtk.vi"("error in (no error)"=w435, "VI Ref (calling VI)"=w432) -> ("error out"=w434:errorcluster, "dup VI Ref"=w431:refnum<vi>)  [unwired: 4 in]
        n149 = disable-structure shown="Disabled" {
          disable-tunnel: w431 -> [w440 _]
          frame Disabled {
            n150 = property class="VI"(reference=w440, "Front Panel.Title"="*VI Title*" ("Front Panel Window:Title")) -> ()  [unwired: 1 in, 2 out]
          }
          frame Enabled {
          }
        }
        n151 = call <vilib>:"Add State(s) to Queue__JKI_lib_State_Machine.vi"("State(s) in (\"\")"=w438) -> ("States Out"=w437:string)  [unwired: 14 in]
      }
      frame "UI: Cursor Set" {
        # "Argument"
        n152 = case shown="\"Idle\", Default" w442 {
          tunnel: w444 -> [w449 w451]
          tunnel: [w448 w450] -> w443
          frame "Idle", Default {
            n153 = call <vilib>:"Unset Busy.vi"("error in (no error)"=w449) -> ("error out"=w448:errorcluster)  [unwired: 10 in]
          }
          frame "Busy" {
            n154 = call <vilib>:"Set Busy.vi"("error in (no error)"=w451) -> ("error out"=w450:errorcluster)  [unwired: 9 in, 1 out]
          }
        }
        n155 = call <vilib>:"Add State(s) to Queue__JKI_lib_State_Machine.vi"("State(s) in (\"\")"=w447) -> ("States Out"=w446:string)  [unwired: 14 in]
      }
      frame "UI: Front Panel State" {
        # "Argument"
        n156 = Unbundle By Name(w455) -> ("Core.Current VI Reference"=w454:refnum<vi>)
        n157 = case shown="\"Open\", Default" w453 {
          tunnel: w457 -> [w463 w476]
          tunnel: [w465 w477] -> w456
          tunnel: w454 -> [w464 w474]
          frame "Open", Default {
            n158 = property class="VI"(reference=w464, error in=w463) -> (reference out=w461:refnum<vi>, error out=w462:errorcluster, "FP.State"=w460:T13)
            n159 = case shown="\"Closed\"" w460 {
              tunnel: [w468 w471] -> w465
              tunnel: w462 -> [w467 w471]
              tunnel: w461 -> [w466 _]
              frame "Closed" {
                n160 = invoke class="VI" method="FP.Open"(reference=w466, error in=w467, "Activate"=TRUE, "State"=T13."Standard") -> (error out=w468:errorcluster)  [unwired: 1 in, 4 out]
              }
              frame "Standard", Default {
              }
            }
          }
          frame "Close" {
            n161 = property class="VI"(reference=w474, error in=w476) -> (reference out=w473:refnum<vi>, error out=w475:errorcluster, "FP.State"=w472:T13)
            n162 = case shown="\"Standard\", \"Hidden\"..\"Maximized\", Default" w472 {
              tunnel: [w478 w481] -> w477
              tunnel: w475 -> [w478 w480]
              tunnel: w473 -> [_ w479]
              frame "Invalid", "Closed" {
              }
              frame "Standard", "Hidden".."Maximized", Default {
                n163 = invoke class="VI" method="FP.Close"(reference=w479, error in=w480) -> (error out=w481:errorcluster)  [unwired: 1 in, 2 out]
              }
            }
          }
        }
        n164 = call <vilib>:"Add State(s) to Queue__JKI_lib_State_Machine.vi"("State(s) in (\"\")"=w459) -> ("States Out"=w458:string)  [unwired: 14 in]
      }
      frame "---------- Macro ----------" {
        n165 = call <vilib>:"Add State(s) to Queue__JKI_lib_State_Machine.vi"("State(s) in (\"\")"=w486) -> ("States Out"=w485:string)  [unwired: 14 in]
      }
      frame "Macro: Initialize" {
        n166 = call <vilib>:"Add State(s) to Queue__JKI_lib_State_Machine.vi"("State(s) in Front (\"\")"=w487, "State(s) in (\"\")"=w492) -> ("States Out"=w491:string)  [unwired: 13 in]
      }
      frame "Macro: Exit" {
        n167 = Unbundle By Name(w500) -> ("Core.Close Panel on Exit?"=w499:bool)
        n168 = Select(t="UI: Front Panel State >> Close", s=w499, f="") -> (s? t:f=w496:string)
        n169 = call <vilib>:"Add State(s) to Queue__JKI_lib_State_Machine.vi"("State(s) in (\"\")"=w496, "State(s) at Back (\"\")"=w493) -> ("States Out"=w495:string)  [unwired: 13 in]
        n170 = call <vilib>:"Add State(s) to Queue__JKI_lib_State_Machine.vi"("State(s) in Front (\"\")"=w495, "State(s) in (\"\")"=w503) -> ("States Out"=w502:string)  [unwired: 13 in]
      }
      frame "-------- API -----------" {
        n171 = call <vilib>:"Add State(s) to Queue__JKI_lib_State_Machine.vi"("State(s) in (\"\")"=w508) -> ("States Out"=w507:string)  [unwired: 14 in]
      }
      frame "API: PrintDitheredImage" {
        n172 = call <vilib>:"Add State(s) to Queue__JKI_lib_State_Machine.vi"("State(s) in (\"\")"=w513) -> ("States Out"=w512:string)  [unwired: 14 in]
      }
      frame "API: InvokePPP" {
        n173 = Unbundle By Name(w518) -> ("Py session"=w526:refnum<k35>, "CuurentSyncTask.vData"=w516:variant)
        n174 = Variant To Data(error in=w524, type=T14 {"product"="", "printer"="", "printhead"=enum."1", "material"="", "weight"=0.0, "density"=0.0, "overprint"=0.0, "print_wt_multiplier"=0.0, "num_of_drops"=0, "gs_source"="", "gs_val_file"=path "", "zone_compensation"=FALSE, "zone_comp_file"=path "", "bitmap"=path "", "save_gs_img"=FALSE, "dithered_save_path"=path "", "gs_save_path"=path "", "rotation"=FALSE, "driver"="", "server"="", "database"="", "user"="", "password"=""} ("PPP_parameters"), Variant=w516) -> (data=w523:T14, error out=w522:errorcluster)
        n175 = call "InvokePPP.vi"("error in (no error)"=w522, "PPP_parameters"=w523, "Py Session"=w526) -> ("error out"=w521:errorcluster, "Cluster"=w515:cluster{"Success":bool, "Status":string}, "Py Session out"=w517:refnum<k35>)  [unwired: 6 in]
        n176 = To Variant(anything=w515) -> (Variant=w514:variant)
        n177 = Bundle By Name(cluster=w518, "CurrentTaskReturnValue"=w514, "Py session"=w517) -> (w519:T3)
        n178 = call <vilib>:"Add State(s) to Queue__JKI_lib_State_Machine.vi"("State(s) in Front (\"\")"="Task: Completed" ("State(s) in Front (\"\")"), "State(s) in (\"\")"=w529) -> ("States Out"=w528:string)  [unwired: 13 in]
      }
      frame "API: SeperateLayersPython" {
        n179 = Unbundle By Name(w550) -> ("Self Reference"=w541:refnum<class "DLP2.lvclass">, "CuurentSyncTask.vData"=w553:variant, "Images"=w543:T1[], "Py session"=w536:refnum<k35>, "ConfigDict"=w531:T11)
        n180 = Variant To Data(error in=w552, type=T16 {"Path_to_Tiff"=path "", "OutputFolder"=path "", "DPI_x"=0, "DPI_y"=0, "Python_Version"=enum."3.9 64"}, Variant=w553) -> (data=w548:T16, error out=w554:errorcluster)
        n181 = Unbundle By Name(w548) -> ("OutputFolder"=w547:path)
        n182 = call "SeperateLayersPython.vi"("error in (no error)"=w554, "Py Session"=w536, "Cluster"=w548) -> ("error out"=w545:errorcluster, "Py Session out"=w535:refnum<k35>, "return value"=w534:cluster{"Success":bool, "Status":string})  [unwired: 6 in]
        n183 = List Folder(path=w547, pattern="*.bmp", error in=w545) -> (path out=w537:path, filenames=w544:string[], error out=w542:errorcluster)  [unwired: 1 in, 1 out]
        n184 = Unbundle By Name(w534) -> ("Success"=→"Split Scale Success":bool)
        n185 = Bundle By Name(cluster=w550, "CurrentTaskReturnValue"=w534, "Py session"=w535) -> (w551:T3)
        n186 = Empty Array?(array=w544) -> (empty?=w533:bool)
        n187 = case shown="False" w533 {
          tunnel: w544 -> [w570 _]
          tunnel: w543 -> [w575 w588]
          tunnel: w537 -> [w574 _]
          tunnel: w542 -> [w568 w587]
          tunnel: [w573 w588] -> w540
          tunnel: [w572 w587] -> w539
          tunnel: w531 -> [w571 _]
          tunnel: [w566 u8[] [] ("Sorted Heads[]")] -> w530
          frame False {
            n188 = call "sortSeprateLayerImagesByAsendingHead.vi"("error in (no error)"=w568, "filenames"=w570, "Data Value Reference in"=w571) -> ("error out"=w567:errorcluster, "filenamesSortedbyAscndingHeads"=w569:string[], "Sorted Heads[]"=w566:u8[])  [unwired: 5 in, 1 out]
            n189 = for {
              tunnel: w569 -> [w585] mode=indexing
              tunnel: w575 -> [w582] mode=indexing
              tunnel: w574 -> [w584]
              shift-right: [w577] -> w572
              shift-left: w567 -> [w581]
              tunnel: [w576] -> w573 mode=indexing
              n190 = Build Path(base path=w584, name or relative path=w585) -> (appended path=w583:path)
              n191 = call "IMAQ ReadFile 2"("File Path"=w583, "error in (no error)"=w581, "Image"=w582) -> ("error out"=w578:errorcluster, "Image Out"=w580:T1)  [unwired: 4 in, 3 out]
              n192 = call "IMAQ Rotate 2"("error in (no error)"=w578, "Angle (degrees)"=0.0, "Image Dst"=w580, "Image Src"=w580) -> ("error out"=w577:errorcluster, "Image Dst Out"=w576:T1)  [unwired: 6 in]
              "ImageMain 2" <- w576
            }
          }
          frame True {
          }
        }
        n193 = case shown="False" w533 {
          tunnel: w541 -> [w564 _]
          tunnel: w540 -> [w563 _]
          tunnel: w539 -> [w562 w565]
          tunnel: [w561 w565] -> w538
          tunnel: w537 -> [w560 _]
          tunnel: w530 -> [w559 _]
          frame False {
            # "Set pvt data and \ntrigger evnt"
            n194 = call "Set SeperatedLayers.vi"("OutputDirPath"=w560, "error in (no error)"=w562, "Sorted Heads[]"=w559, "Images"=w563, "DLP2 in"=w564) -> ("error out"=w561:errorcluster)  [unwired: 5 in, 1 out]
          }
          frame True {
          }
        }
        n195 = call <vilib>:"Add State(s) to Queue__JKI_lib_State_Machine.vi"("State(s) in Front (\"\")"="Task: Completed" ("State(s) in Front (\"\")"), "State(s) in (\"\")"=w558) -> ("States Out"=w557:string)  [unwired: 13 in]
      }
      frame "API: LoadImages" {
        n196 = Unbundle By Name(w603) -> ("Self Reference"=w598:refnum<class "DLP2.lvclass">, "CuurentSyncTask.vData"=w605:variant, "Images"=w599:T1[])
        n197 = Variant To Data(error in=w604, type=T18 {"Images[]"=[], "Calibration"=FALSE, "Heads[]"=[]} ("LoadImagesData"), Variant=w605) -> (data=w601:T18, error out=w593:errorcluster)
        n198 = Unbundle By Name(w601) -> ("Heads[]"=w590:u8[], "Calibration"=w591:bool, "Images[]"=w592:path[])
        n199 = Empty Array?(array=w592) -> (empty?=w600:bool)
        n200 = case shown="False" w600 {
          tunnel: w599 -> [w616 w656]
          tunnel: w592 -> [w615 _]
          tunnel: w593 -> [w614 w655]
          tunnel: [w613 w656] -> w597
          tunnel: [w612 w655] -> w596
          tunnel: w591 -> [w611 _]
          tunnel: w590 -> [w610 w654]
          tunnel: [w609 w654] -> w589
          frame False {
            n201 = for {
              tunnel: w616 -> [w626] mode=indexing
              tunnel: w615 -> [w622] mode=indexing
              tunnel: [w623] -> w613 mode=indexing if=w617
              tunnel: w611 -> [w620]
              tunnel: w614 -> [w625]
              tunnel: [w624] -> w612
              tunnel: w610 -> [w619] mode=indexing
              tunnel: [w618] -> w609 mode=indexing if=w617
              n202 = call-poly <userlib>:"File Exists__ogtk.vi"("file path"=w622) -> ("exists"=w621:bool)  [unwired: 6 in, 1 out]
              n203 = case shown="True" w621 {
                selector: w621 -> [w630 w634]
                tunnel: w626 -> [w629 w640]
                tunnel: w625 -> [w628 w639]
                tunnel: [w628 w636] -> w624
                tunnel: [w629 w633] -> w623
                tunnel: w622 -> [_ w635]
                tunnel: [w630 w634] -> w617
                tunnel: w620 -> [_ w632]
                tunnel: w619 -> [w627 w631]
                tunnel: [w627 w631] -> w618
                frame False {
                }
                frame True {
                  n204 = call "IMAQ ReadFile 2"("File Path"=w635, "error in (no error)"=w639, "Image"=w640) -> ("error out"=w637:errorcluster, "Image Out"=w638:T1)  [unwired: 4 in, 3 out]
                  n205 = case shown="False" w632 {
                    tunnel: w638 -> [w644 w653]
                    tunnel: w637 -> [w643 w651]
                    tunnel: [w642 w647] -> w636
                    tunnel: [w641 w650] -> w633
                    tunnel: w631 -> [_ _]
                    frame False {
                      n206 = call "IMAQ Rotate 2"("error in (no error)"=w643, "Angle (degrees)"=0.0, "Image Dst"=w644, "Image Src"=w644) -> ("error out"=w642:errorcluster, "Image Dst Out"=w641:T1)  [unwired: 6 in]
                    }
                    frame True {
                      n207 = call "IMAQ Rotate 2"("Maintain Size"=FALSE, "error in (no error)"=w651, "Angle (degrees)"=90.0, "Image Dst"=w653, "Image Src"=w653) -> ("error out"=w648:errorcluster, "Image Dst Out"=w646:T1)  [unwired: 5 in]
                      n208 = call "IMAQ Inverse"("error in (no error)"=w648, "Image Mask"=w646, "Image Src"=w646) -> ("error out"=w647:errorcluster, "Image Dst Out"=w650:T1)  [unwired: 7 in]
                    }
                  }
                  "ImageMain 3" <- w633
                }
              }
            }
          }
          frame True {
          }
        }
        n209 = call <vilib>:"Add State(s) to Queue__JKI_lib_State_Machine.vi"("State(s) in Front (\"\")"="Task: Completed" ("State(s) in Front (\"\")"), "State(s) in (\"\")"=w608) -> ("States Out"=w607:string)  [unwired: 13 in]
        n210 = call "Set SeperatedLayers.vi"("error in (no error)"=w596, "Sorted Heads[]"=w589, "Images"=w597, "DLP2 in"=w598) -> ("error out"=w595:errorcluster)  [unwired: 6 in, 1 out]
      }
      frame "API: LoadTiffImage" {
        n211 = Unbundle By Name(w663) -> ("CuurentSyncTask.vData"=w662:variant)
        n212 = Variant To Data(error in=w661, type=path "", Variant=w662) -> (error out=w658:errorcluster)  [unwired: 1 out]
        n213 = Bundle By Name(cluster=w663, "CurrentTaskReturnValue"=variant) -> (w660:T3)
        n214 = call <vilib>:"Add State(s) to Queue__JKI_lib_State_Machine.vi"("State(s) in Front (\"\")"="Task: Completed" ("State(s) in Front (\"\")"), "State(s) in (\"\")"=w667) -> ("States Out"=w666:string)  [unwired: 13 in]
      }
      frame "---------- Action ----------" {
        n215 = call <vilib>:"Add State(s) to Queue__JKI_lib_State_Machine.vi"("State(s) in (\"\")"=w672) -> ("States Out"=w671:string)  [unwired: 14 in]
      }
      frame "Action: Wait" {
        n216 = Scan From String(format string="%d", input string=w673, error in=w675, default 1=u32 0) -> (error out=w679:errorcluster, output 1=w678:u32)  [unwired: 1 in, 2 out]
        n217 = call <userlib>:"Wait (ms)__ogtk.vi"("error in (no error)"=w679, "milliseconds to wait"=w678) -> ("error out"=w674:errorcluster)  [unwired: 8 in, 1 out]
        n218 = call <vilib>:"Add State(s) to Queue__JKI_lib_State_Machine.vi"("State(s) in (\"\")"=w683) -> ("States Out"=w682:string)  [unwired: 14 in]
      }
      frame "Action: Terminate AsyncLoop" {
        n219 = Unbundle By Name(w689) -> ("SMQ"=w688:refnum<queue>)
        n220 = Flush Queue(queue=w688) -> (queue out=w687:refnum<queue>)  [unwired: 1 in, 2 out]
        n221 = call <vilib>:"Add State to Queue with vData.vi"("queue in"=w687, "state in"="Macro: Exit", "error in"=w685) -> ("error out"=w684:errorcluster)  [unwired: 9 in, 3 out]
        n222 = call <vilib>:"Add State(s) to Queue__JKI_lib_State_Machine.vi"("State(s) in (\"\")"=w692) -> ("States Out"=w691:string)  [unwired: 14 in]
      }
      frame "---------- Tasks -----------" {
        n223 = call <vilib>:"Add State(s) to Queue__JKI_lib_State_Machine.vi"("State(s) in (\"\")"=w697) -> ("States Out"=w696:string)  [unwired: 14 in]
      }
      frame "Task: Remove on Error" {
        n224 = Unbundle By Name(w699) -> ("Public Events.API Return Event"=w705:refnum<user-event>, "Tasks"=w704:T7[])
        n225 = for {
          tunnel: w705 -> [w715]
          tunnel: w704 -> [w714] mode=indexing
          shift-right: [w710] -> w703
          shift-left: w702 -> [w711]
          n226 = Get Date/Time In Seconds() -> (seconds since 1Jan1904=w712:timestamp)
          n227 = Bundle By Name(cluster=w714, "Task.Task State"=TD_Sync_API_Task_State."Errored", "Task.Time Stamp"=w712) -> (w713:T7)
          n228 = Generate User Event(user event=w715, event data cluster=w713, error in=w711) -> (error out=w710:errorcluster)  [unwired: 1 in, 1 out]
        }
        n229 = Bundle By Name(cluster=w699, "TO"=-1, "Tasks"=T7[] []) -> (w700:T3)
        n230 = call <vilib>:"Add State(s) to Queue__JKI_lib_State_Machine.vi"("State(s) in (\"\")"=w708) -> ("States Out"=w707:string)  [unwired: 14 in]
      }
      frame "Task: Check Pending" {
        n231 = Unbundle By Name(w717) -> ("Public Events.API Executed Event"=w723:refnum<user-event>, "Task Start ms"=w722:u32, "Tasks"=w721:T7[])
        n232 = Empty Array?(array=w721) -> (empty?=w724:bool)
        n233 = case shown="False" w724 {
          tunnel: w723 -> [_ _]
          tunnel: w719 -> [w738 w744]
          tunnel: [w736 w744] -> w720
          tunnel: w722 -> [_ _]
          tunnel: w721 -> [w742 _]
          tunnel: [w735 _] -> w716
          tunnel: w717 -> [w734 w743]
          tunnel: [w732 w743] -> w718
          frame False {
            n234 = Index Array(array=w742) -> (element=w740:T7)  [unwired: 1 in]
            n235 = Unbundle By Name(w740) -> ("Command"=w739:variant)
            n236 = Variant To Data(error in=w738, type=T10 {"Time Stamp"=timestamp(0 s since 1904-01-01), "CmdMsg"="", "vData"=variant} ("Async EvData"), Variant=w739) -> (data=w729:T10, error out=w737:errorcluster)
            n237 = Tick Count (ms)() -> (millisecond timer value=w733:u32)
            n238 = Unbundle By Name(w729) -> ("CmdMsg"=w728:string)
            n239 = Bundle By Name(cluster=w734, "TO"=100, "Task Start ms"=w733, "CuurentSyncTask"=w729) -> (w732:T3)
            n240 = Format Into String(format string="API: %s", error in=w737, w728) -> (resulting string=w735:string, error out=w736:errorcluster)  [unwired: 1 in]
          }
          frame True {
          }
        }
        n241 = call <vilib>:"Add State(s) to Queue__JKI_lib_State_Machine.vi"("State(s) in Front (\"\")"=w716, "State(s) in (\"\")"=w727) -> ("States Out"=w726:string)  [unwired: 13 in]
      }
      frame "Task: Check Timeout" {
        n242 = Unbundle By Name(w747) -> ("Public Events.API Executed Event"=w751:refnum<user-event>, "Task Start ms"=w748:u32, "Tasks"=w750:T7[])
        n243 = Index Array(array=w750) -> (element=w749:T7)  [unwired: 1 in]
        n244 = Empty Array?(array=w750) -> (empty?=w752:bool)
        n245 = case shown="False" w752 {
          tunnel: w751 -> [w758 _]
          tunnel: w745 -> [w763 w772]
          tunnel: [w759 w772] -> w746
          tunnel: w749 -> [w762 _]
          tunnel: w748 -> [w766 _]
          frame False {
            n246 = Unbundle By Name(w762) -> ("Task.Timeout (ms)"=w764:u32)
            n247 = Tick Count (ms)() -> (millisecond timer value=w757:u32)
            n248 = Subtract(x=w757, y=w766) -> (x-y=w765:u32)
            n249 = Bundle By Name(cluster=w762, "Task.Task State"=TD_Sync_API_Task_State."Errored") -> (w761:T7)
            n250 = Greater Or Equal?(x=w765, y=w764) -> (x >= y?=w760:bool)
            n251 = case shown="True" w760 {
              tunnel: w763 -> [w767 w771]
              tunnel: w761 -> [_ w769]
              tunnel: [w767 w770] -> w759
              tunnel: w758 -> [_ w768]
              frame False {
              }
              frame True {
                n252 = Generate User Event(user event=w768, event data cluster=w769, error in=w771) -> (error out=w770:errorcluster)  [unwired: 1 in, 1 out]
              }
            }
          }
          frame True {
          }
        }
        n253 = call <vilib>:"Add State(s) to Queue__JKI_lib_State_Machine.vi"("State(s) in (\"\")"=w755) -> ("States Out"=w754:string)  [unwired: 14 in]
      }
      frame "Task: Completed" {
        n254 = Unbundle By Name(w775) -> ("Public Events.API Executed Event"=w778:refnum<user-event>, "Tasks"=w777:T7[], "CurrentTaskReturnValue"=w776:variant)
        n255 = Empty Array?(array=w777) -> (empty?=w779:bool)
        n256 = case shown="False" w779 {
          tunnel: w778 -> [w788 _]
          tunnel: w777 -> [w789 _]
          tunnel: w773 -> [w787 w790]
          tunnel: [w786 w790] -> w774
          tunnel: w776 -> [w783 _]
          frame False {
            n257 = Index Array(array=w789) -> (element=w785:T7)  [unwired: 1 in]
            n258 = Bundle By Name(cluster=w785, "Return Value"=w783) -> (w784:T7)
            n259 = Generate User Event(user event=w788, event data cluster=w784, error in=w787) -> (error out=w786:errorcluster)  [unwired: 1 in, 1 out]
          }
          frame True {
          }
        }
        n260 = call <vilib>:"Add State(s) to Queue__JKI_lib_State_Machine.vi"("State(s) in (\"\")"=w782) -> ("States Out"=w781:string)  [unwired: 14 in]
      }
    }
  }
  n261 = Merge Errors(w4, w3) -> ()  [unwired: 1 out]
